vi "EnabledChannelsEnumDisable.vi"(10 "Number Enabled":dbl, 11 "Enum in":refnum<vi>) -> ()   [LabVIEW 2026]
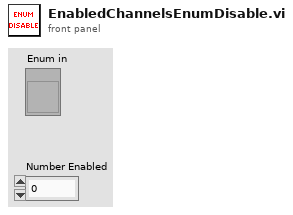
[diagram p1: front panel]
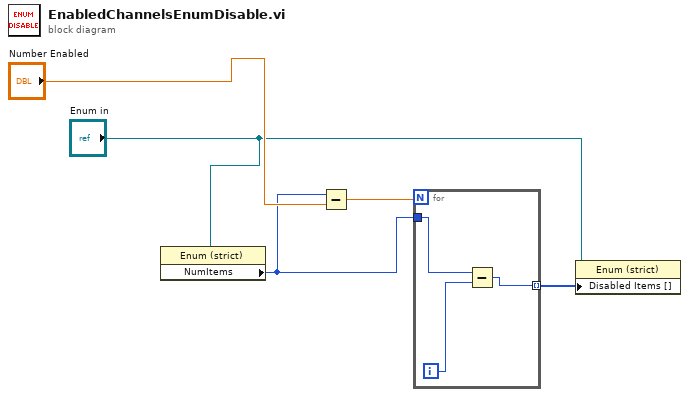
[diagram p0: block diagram]
diagram:
  n1 = property class="Enum (strict)"(reference="Enum in") -> ("NumItems"=w4:u32)  [unwired: 1 in, 2 out]
  n2 = Subtract(x=w4, y="Number Enabled") -> (x-y=w1:dbl)
  n3 = for {
    N: w1 -> [_]
    tunnel: w4 -> [w8]
    tunnel: [w6] -> w3 mode=indexing
    i -> [w7]
    n4 = Subtract(x=w8, y=w7) -> (x-y=w6:u32)
  }
  n5 = property class="Enum (strict)"(reference="Enum in", "Disabled Items []"=w3) -> ()  [unwired: 1 in, 2 out]
